vi "中文字符显示实验.vi"() -> ()   [LabVIEW 2011]
uses:
  <vilib>/STM32_DriverVI_Interface_F4/LCD/Show_Mode_F4.ctl
  <vilib>/STM32_DriverVI_Interface_F4/LCD/Font_Size_F4.ctl
  <vilib>/STM32_DriverVI_Interface_F4/LCD/Brush Color_Index_F4.ctl
  <vilib>/STM32_DriverVI_Interface_F4/LCD/LCD_Init_F4.vi
panel:
  out "Update_Success?":bool
  in  "fresh":bool
  out "Init_Success?":bool
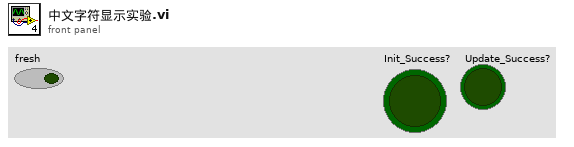
[diagram p1: front panel]
types:
  T1 = enum8{"P0", "P1", "P2", "P3", "P4", "P5", "P6", "P7", "P8", "P9", "P10", "P11", "P12", "P13", "P14", "P15"}
  T2 = enum8{"Port_A", "Port_B", "Port_C", "Port_D", "Port_E", "Port_F", "Port_G", "Port_H", "Port_I"}
  T3 = typedef "Show_Mode_F4.ctl" = enum8{"非叠加显示", "叠加显示"}
  T4 = typedef "Font_Size_F4.ctl" = enum8{"Small_Font（12）", "Big_Font（16）"}
  T5 = typedef "Brush Color_Index_F4.ctl" = enum8{"White", "Black", "Blue", "Green_Blue", "Red", "Magenta（品红）", "Green", "Cyan（青色）", "Yellow", "Brown", "Brown_Red", "Gray", "Dark_Blue", "Light_Blue", "Gray_Blue", "Light_Green", "Light_Gray", "Light_Gray_Blue", "Light_Brown_Blue"}
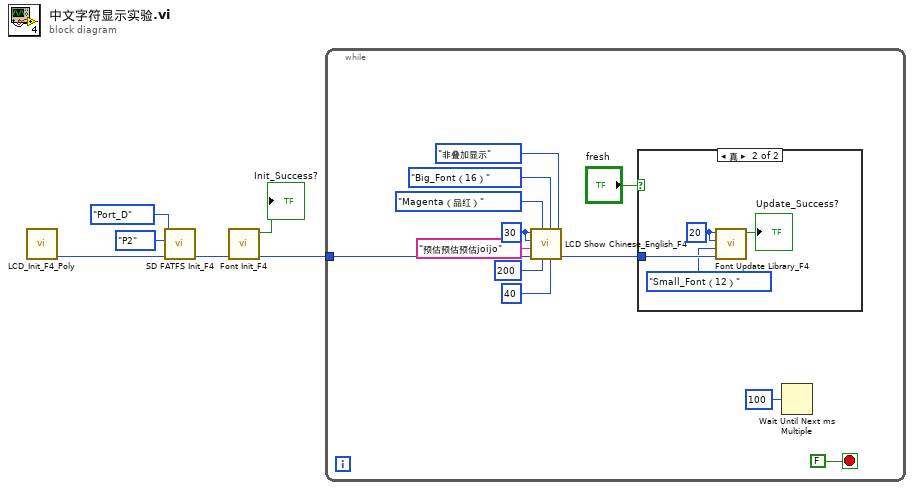
[diagram p0: block diagram]
diagram:
  n1 = call-poly <vilib>:"LCD_Init_F4_Poly.vi"() -> ("err_out"=w6:u8)  [unwired: 10 in, 1 out]
  n2 = call <vilib>:"SD FATFS Init_F4.vi"("err_in"=w6, "SD_CS_pin"=T1."P2", "SD_CS_PortX"=T2."Port_D") -> ("err_out"=w3:u8)  [unwired: 7 in, 1 out]
  n3 = call <vilib>:"Font Init_F4.vi"("err_in"=w3) -> ("err_out"=w1:u8, "Init_Success?"=→"Init_Success?":bool)  [unwired: 9 in]
  n4 = while {
    tunnel: w1 -> [w18]
    stop <- FALSE stop-if-true
    w17 = u16 30 ("X_Position")
    n5 = call <vilib>:"LCD Show Chinese_English_F4.vi"("Show_Mode"=Show_Mode_F4."非叠加显示", "Height"=u16 40, "Font_Size"=Font_Size_F4."Big_Font（16）", "Width"=u16 200, "Brush Color"=Brush_Color_Index_F4."Magenta（品红）", "err_in"=w18, "String"="预估预估预估joijo", "Y_Position"=w17, "X_Position"=w17) -> ("err_out"=w9:u8)  [unwired: 2 in]
    n6 = case shown="真" "fresh" {
      tunnel: w9 -> [_ w22]
      frame False {
      }
      frame True {
        w21 = u16 20 ("X_Position")
        n7 = call <vilib>:"Font Update Library_F4.vi"("err_in"=w22, "Font_Size"=Font_Size_F4."Small_Font（12）", "Y_Position"=w21, "X_Position"=w21) -> ("Update_Success?"=→"Update_Success?":bool)  [unwired: 6 in, 1 out]
      }
    }
    n8 = Wait Until Next ms Multiple(millisecond multiple=u32 100 ("毫秒倍数")) -> ()  [unwired: 1 out]
  }
